vi "Timeout.vi"(0 "reference in":refnum<class "TimedDoor.lvclass">, 1 "TimeoutID":u32, 2 "TimeoutName":string, 5 "error in (no error)":errorcluster) -> (14 "reference out":refnum<class "TimedDoor.lvclass">, 19 "error out":errorcluster)   [LabVIEW 2020, in "TimedDoor.lvclass"]
uses:
  TimedDoor.lvclass
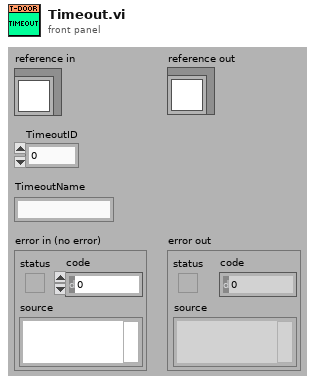
[diagram p1: front panel]
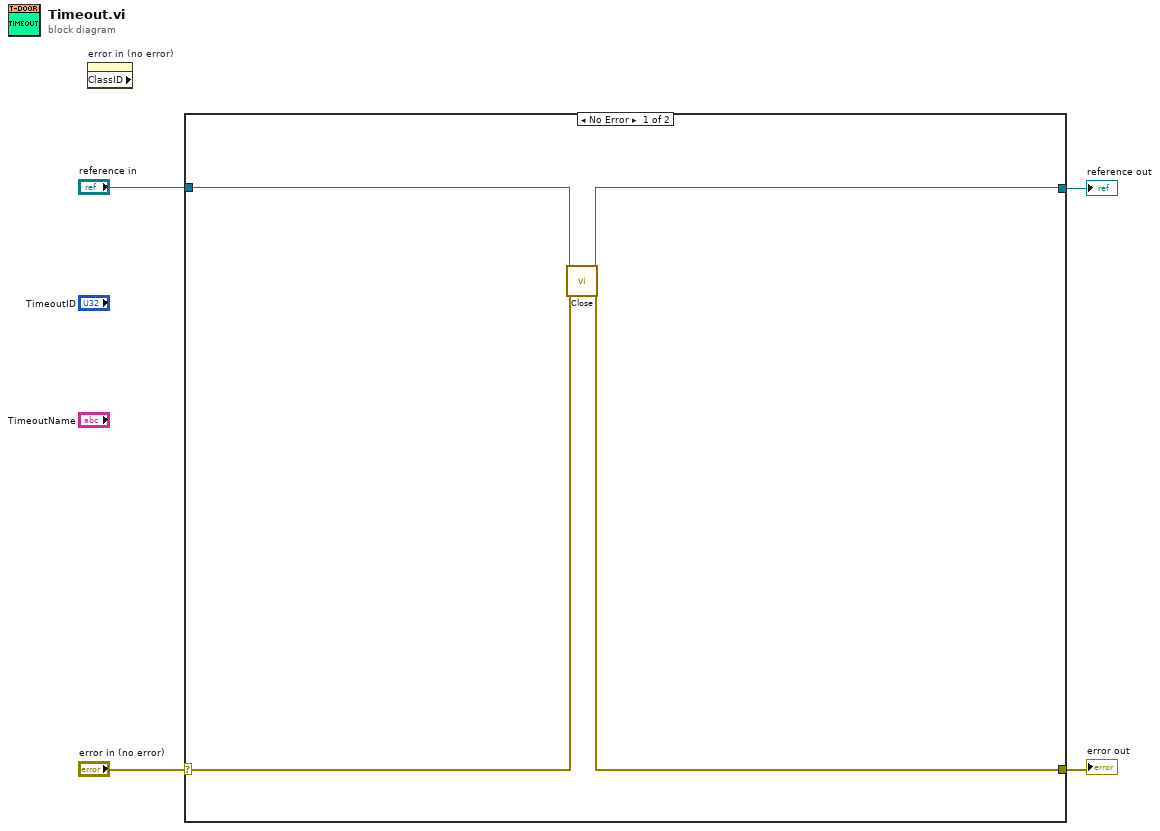
[diagram p0: block diagram]
diagram:
  n1 = property on="error in (no error)" class="Clust (strict)" props=["ClassID"]() -> ()  [unwired: 2 in, 3 out]
  n2 = case shown="No Error" "error in (no error)" {
    selector: "error in (no error)" -> [w6 w10]
    tunnel: [w5 w10] -> w3
    tunnel: [w7 w9] -> w1
    tunnel: "reference in" -> [w8 w9]
    frame No Error {
      n3 = call-dynamic "Close.vi"("reference in"=w8, "error in (no error)"=w6) -> ("reference out"=w7:refnum<class "TimedDoor.lvclass">, "error out"=w5:errorcluster)  [unwired: 16 in]
    }
    frame Error {
    }
  }
  "error out" <- w3
  "reference out" <- w1
